vi "check odor config array value errors (sub-vi).vi"(7 "manifold configuration array":T5, 10 "odor config array":T1) -> (4 "value error":errorcluster)   [LabVIEW 2021]
uses:
  type-defs/manifold configuration cluster array (type def).ctl
  type-defs/manifold configuration cluster (type def).ctl
  type-defs/manifold selection.ctl
  type-defs/single port single odor cluster.ctl
  type-defs/port number (type def).ctl
  type-defs/odor selection (type def).ctl
  type-defs/odor color (type def).ctl
  type-defs/odor description array (type def).ctl
  type-defs/odor info cluster (type def).ctl
  aaae10a4-c4df-4c94-bb8f-667a836e8f9b.vi
  <vilib>/ErrorRing/Error Ring.xnode
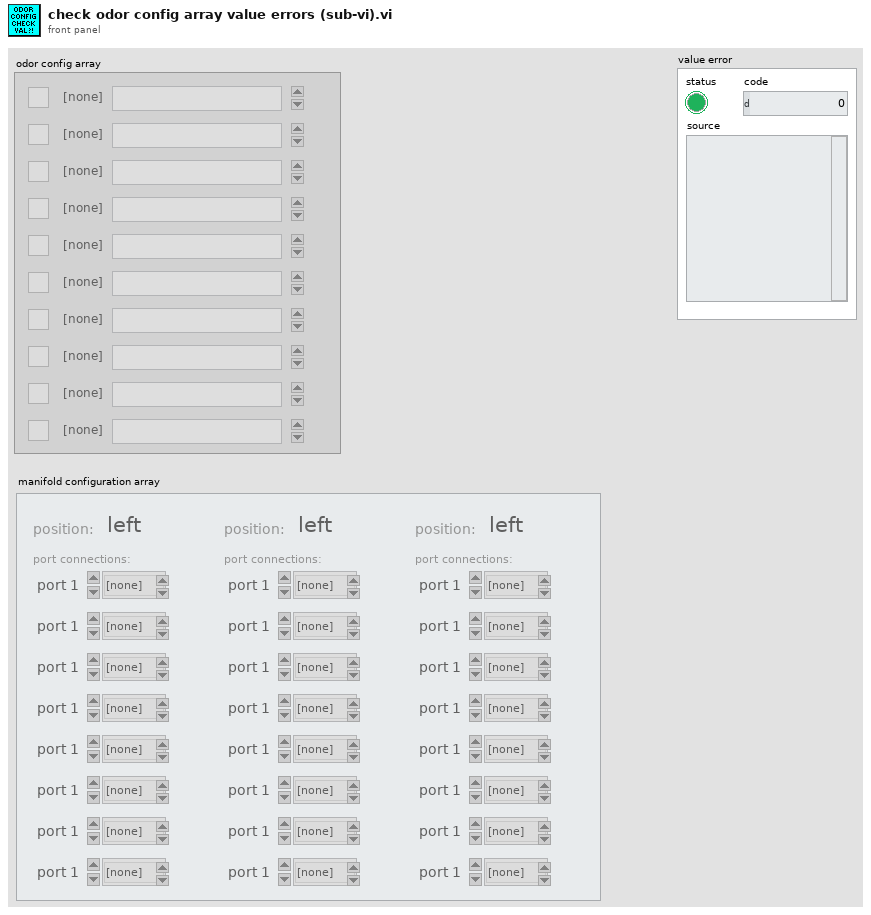
[diagram p1: front panel]
types:
  T1 = typedef "odor description array (type def).ctl" = T2[]
  T2 = typedef "odor info cluster (type def).ctl" = cluster{"odor channel":T3, "odor description":string, "odor color":T4, "odor channel active":bool}
  T3 = typedef "odor selection (type def).ctl" = enum16{"[none]", "odor 1", "odor 2", "odor 3", "odor 4", "odor 5", "odor 6", "odor 7", "odor 8", "odor 9", "odor 10"}
  T4 = typedef "odor color (type def).ctl" = u16
  T5 = typedef "manifold configuration cluster array (type def).ctl" = T6[]
  T6 = typedef "manifold configuration cluster (type def).ctl" = cluster{"position:":T7, "port connections:":T8[]}
  T7 = typedef "manifold selection.ctl" = enum16{"left", "middle", "right"}
  T8 = typedef "single port single odor cluster.ctl" = cluster{"port number":T9, "connected odor":T3, "error":bool, "odor color":T4}
  T9 = typedef "port number (type def).ctl" = enum16{"port 1", "port 2", "port 3", "port 4", "port 5", "port 6", "port 7", "port 8"}
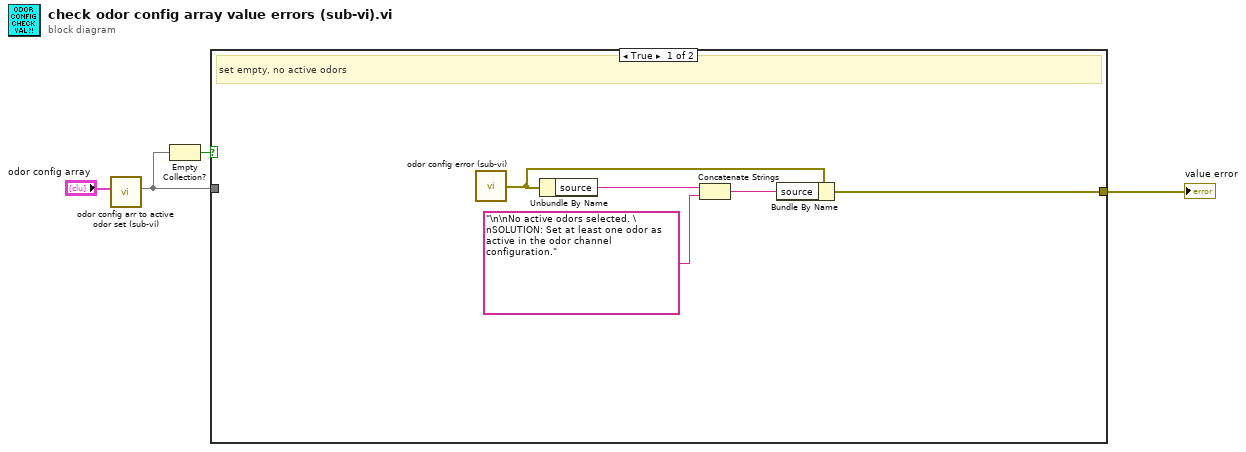
[diagram p0: block diagram]
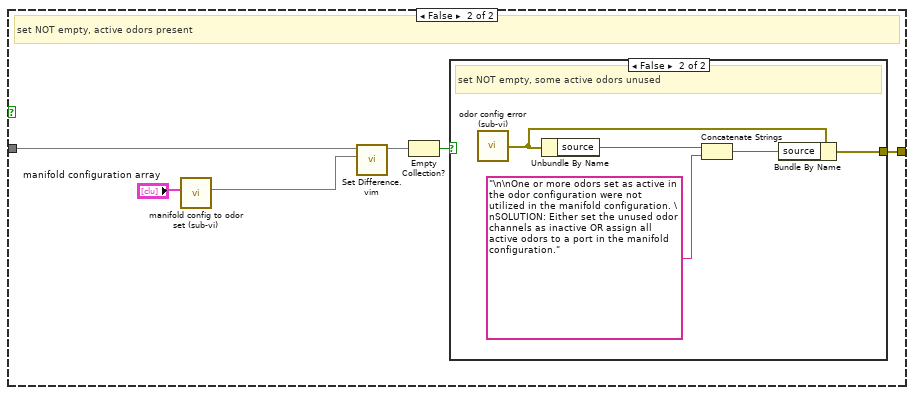
[diagram p2: hidden frame]
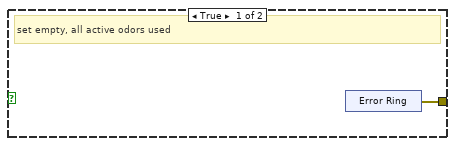
[diagram p3: hidden frame]
diagram:
  n1 = call "odor config arr to active odor set (sub-vi).vi"("odor descriptions"="odor config array") -> ("active odor chanel set"=w3:set{T3})  [unwired: 10 in]
  n2 = Empty Collection?(1:w3) -> (0:w2:bool)
  n3 = case shown="True" w2 {
    tunnel: w3 -> [_ w11]
    tunnel: [w5 w10] -> w1
    frame True {
      # "set empty, no active odors"
      n4 = call "odor config error (sub-vi).vi"() -> ("error"=w9:errorcluster)  [unwired: 1 in]
      n5 = Unbundle By Name(w9) -> ("source"=w8:string)
      n6 = Concatenate Strings(w8, "\n\nNo active odors selected. \nSOLUTION: Set at least one odor as active in the odor channel configuration." ("string")) -> (w7:string)
      n7 = Bundle By Name(cluster=w9, "source"=w7) -> (w5:errorcluster)
    }
    frame False {
      # "set NOT empty, active odors present"
      n8 = call "manifold config to odor set (sub-vi).vi"("manifold configuration"="manifold configuration array") -> ("utilized odor set"=w14:set{T3})  [unwired: 10 in]
      n9 = call "Set Difference.vim"("set 2"=w14, "set 1"=w11) -> ("difference"=w13:set{T3})  [unwired: 9 in]
      n10 = Empty Collection?(1:w13) -> (0:w12:bool)
      n11 = case shown="False" w12 {
        tunnel: [w16 w21] -> w10
        frame True {
          # "set empty, all active odors used"
          n12 = xnode "Error Ring"() -> ("error out"=w16:errorcluster)
        }
        frame False {
          # "set NOT empty, some active odors unused"
          n13 = call "odor config error (sub-vi).vi"() -> ("error"=w22:errorcluster)  [unwired: 1 in]
          n14 = Unbundle By Name(w22) -> ("source"=w20:string)
          n15 = Concatenate Strings(w20, "\n\nOne or more odors set as active in the odor configuration were not utilized in the manifold configuration. \nSOLUTION: Either set the unused odor channels as inactive OR assign all active odors to a port in the manifold configuration." ("string")) -> (w19:string)
          n16 = Bundle By Name(cluster=w22, "source"=w19) -> (w21:errorcluster)
        }
      }
    }
  }
  "value error" <- w1
